vi "NT_LL_Write Boolean.vi"(8 "error in (no error)":errorcluster, 9 "Boolean":bool, 10 "timestamp":u64, 11 "publishHandle":u32) -> (0 "error out":errorcluster, 3 "success":u32)   [LabVIEW 2025]
uses:
  ntcoreffi.dll
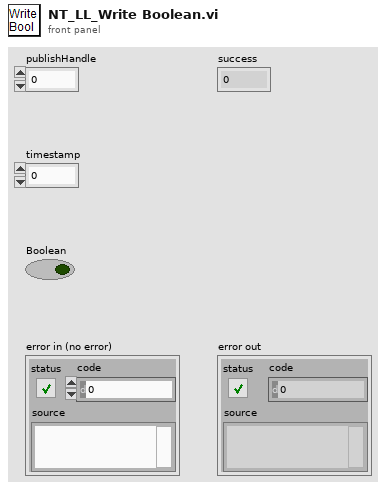
[diagram p1: front panel]
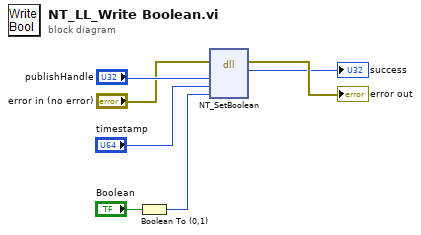
[diagram p0: block diagram]
diagram:
  n1 = Boolean To (0,1)(Boolean="Boolean") -> (0, 1=w1:i16)
  n2 = dll-call lib="ntcoreffi.*" fn="NT_SetBoolean"(error in="error in (no error)", "publishHandle"="publishHandle", "time"="timestamp", "value"=w1) -> (error out=→"error out":errorcluster, "success"=→"success":u32)  [unwired: 5 in, 1 out]
